vi "Load Settings from XML.vi"(8 "error in (no error)":errorcluster, 11 "Settings In":T2) -> (0 "error out":errorcluster, 3 "Settings Out":T2)   [LabVIEW 2025, in "Settings.lvlib"]
doc: "Attempts to load previous user specified settings from an XML file.\n\nThis VI will not generate an error. If a suitable XML file can't be loaded and parsed then it will simply return the default settings."
uses:
  Settings.lvlib
  Settings.ctl
  Acquisition/Acquistion_Configuration.ctl
  Acquisition/Signal Type.ctl
  Logging/Logging Configuration.ctl
  <vilib>/Utility/xml.llb/Read From XML File(string).vi
  <vilib>/Utility/xml.llb/Write to XML File(string).vi
  Acquisition/Acquisition.lvlib
  Logging/Logging.lvlib
panel:
  in  "Logging Configuration":T1
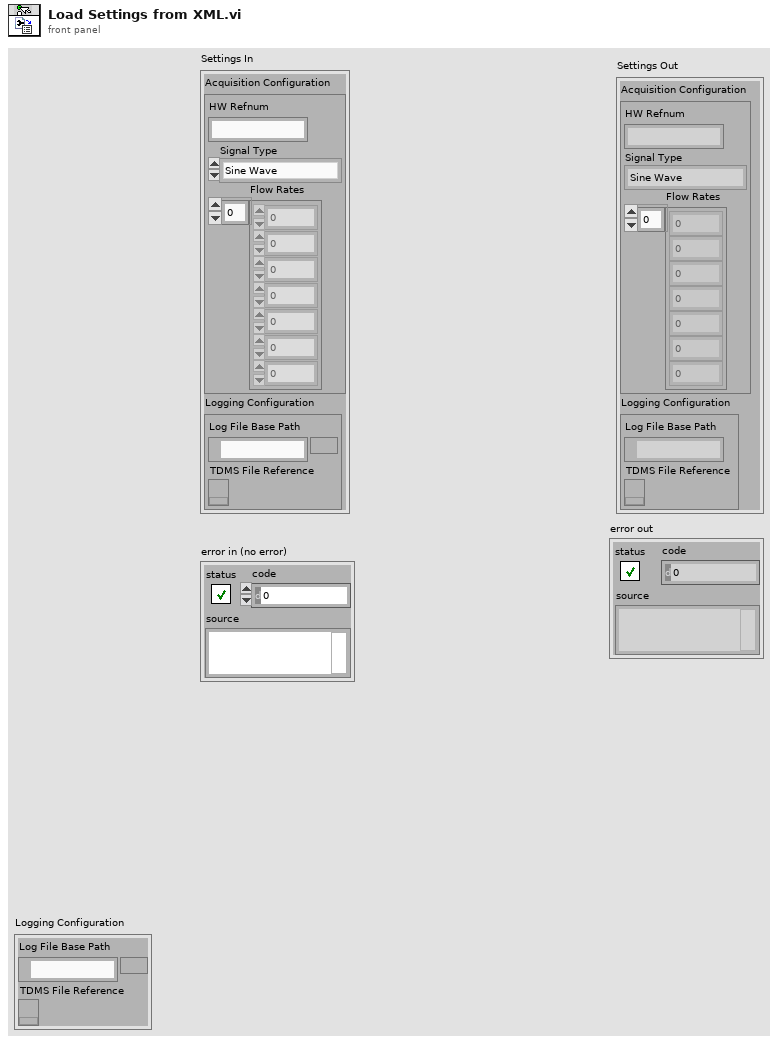
[diagram p1: front panel]
types:
  T1 = typedef "Logging.lvlib/Logging Configuration.ctl" = cluster{"Log File Base Path":path, "TDMS File Reference":refnum<k34>}
  T2 = typedef "Settings.lvlib/Settings.ctl" = cluster{"Acquisition Configuration":T3, "Logging Configuration":T1}
  T3 = typedef "Acquisition.lvlib/Acquistion_Configuration.ctl" = cluster{"HW Refnum":string, "Signal Type":T4, "Flow Rates":dbl[]}
  T4 = typedef "Acquisition.lvlib/Signal Type.ctl" = enum16{"Sine Wave", "Square with Noise"}
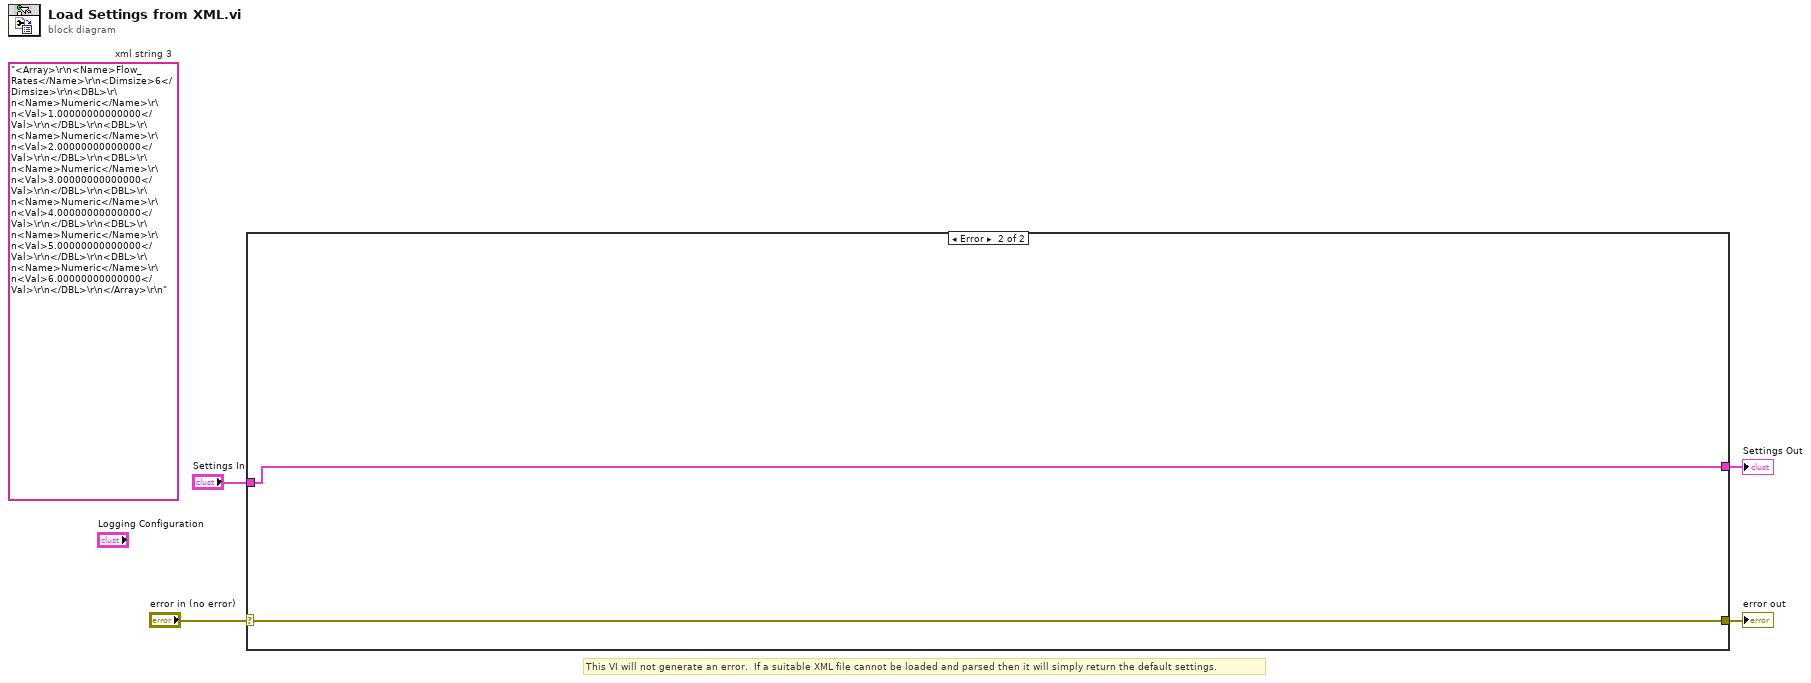
[diagram p0: block diagram]
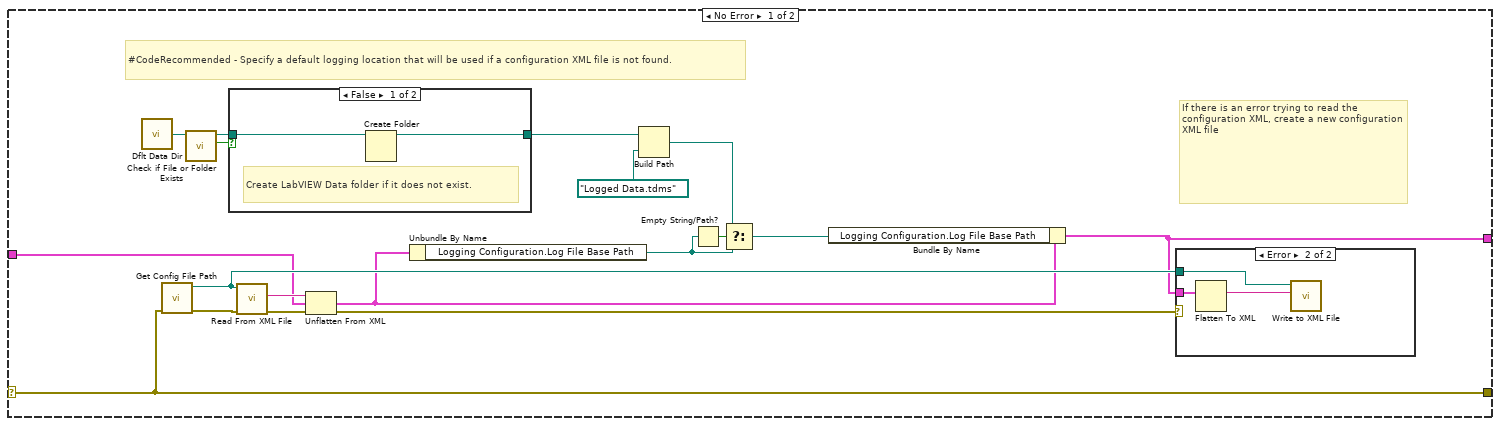
[diagram p2: hidden frame]
diagram:
  (unwired) "<Array>\r\n<Name>Flow_Rates</Name>\r\n<Dimsize>6</Dimsize>\r\n<DBL>\r\n<Name>Numeric</Name>\r\n<Val>1.00000000000000</Val>\r\n</DBL>\r\n<DBL>\r\n<Name>Numeric</Name>\r\n<Val>2.00000000000000</Val>\r\n</DBL>\r\n<DBL>\r\n<Name>Numeric</Name>\r\n<Val>3.00000000000000</Val>\r\n</DBL>\r\n<DBL>\r\n<Name>Numeric</Name>\r\n<Val>4.00000000000000</Val>\r\n</DBL>\r\n<DBL>\r\n<Name>Numeric</Name>\r\n<Val>5.00000000000000</Val>\r\n</DBL>\r\n<DBL>\r\n<Name>Numeric</Name>\r\n<Val>6.00000000000000</Val>\r\n</DBL>\r\n</Array>\r\n"  # xml string 3
  # "This VI will not generate an error.  If a suitable XML file cannot be loaded and parsed then it will simply return the default settings."
  n1 = case shown="Error" "error in (no error)" {
    selector: "error in (no error)" -> [w21 w30]
    tunnel: [w21 w30] -> w4
    tunnel: [w6 w29] -> w2
    tunnel: "Settings In" -> [w5 w29]
    frame No Error {
      # "If there is an error trying to read the configuration XML, create a new configuration XML file"
      # "#CodeRecommended - Specify a default logging location that will be used if a configuration XML file is not found."
      n2 = call <vilib>:"Dflt Data Dir.vi"() -> ("App:Default Data Directory"=w15:path)
      n3 = call "Get Config File Path.vi"("error in (no error)"=w21) -> ("error out"=w22:errorcluster, "XML File Path"=w19:path)  [unwired: 9 in]
      n4 = call <vilib>:"Check if File or Folder Exists.vi"("path"=w15) -> ("file or folder exists?"=w14:bool, "dup path"=w13:path)  [unwired: 8 in, 1 out]
      n5 = case shown="False" w14 {
        tunnel: w13 -> [w24 w25]
        tunnel: [w23 w25] -> w12
        frame False {
          # "Create LabVIEW Data folder if it does not exist."
          n6 = Create Folder(path (use dialog)=w24) -> (created path=w23:path)  [unwired: 2 in, 2 out]
        }
        frame True {
        }
      }
      n7 = call-poly <vilib>:"Read From XML File.vi"("error in (no error)"=w22, "XML File Path"=w19) -> ("error out"=w18:errorcluster, "XML Elements"=w11:string)  [unwired: 7 in, 1 out]
      n8 = Unflatten From XML(xml string=w11, type=w5, error in (no error)=w18) -> (value=w7:T2, error out=w17:errorcluster)
      n9 = Unbundle By Name(w7) -> ("Logging Configuration.Log File Base Path"=w9:path)
      n10 = Build Path(base path=w12, name or relative path=path "Logged Data.tdms" ("App:Default Data Directory")) -> (appended path=w16:path)
      n11 = Empty String/Path?(string/path=w9) -> (empty?=w10:bool)
      n12 = Select(t=w16, s=w10, f=w9) -> (s? t:f=w8:path)
      n13 = Bundle By Name(cluster=w7, "Logging Configuration.Log File Base Path"=w8) -> (w6:T2)
      n14 = case shown="Error" w17 {
        tunnel: w6 -> [_ w28]
        tunnel: w19 -> [_ w26]
        frame No Error {
        }
        frame Error {
          n15 = Flatten To XML(6:w28) -> (2:w27:string)
          n16 = call-poly <vilib>:"Write to XML File.vi"("XML Input"=w27, "XML File Path"=w26) -> ()  [unwired: 7 in, 3 out]
        }
      }
    }
    frame Error {
    }
  }
  "error out" <- w4
  "Settings Out" <- w2
